vi "Set PublicEvents.vi"(8 "error in (no error)":errorcluster, 10 "Public Events":T1, 11 "DbgTimers in":refnum<class "DbgTimers.lvclass">) -> (0 "error out":errorcluster, 3 "DbgTimers out":refnum<class "DbgTimers.lvclass">)   [LabVIEW 2017, in "DbgTimers.lvclass"]
doc: "Developed by Kevin Thompson\nkevin@thompsonengineering.net\n\nCopyright 2018-2020\nThompson Engineering, LLC"
uses:
  DbgTimers.lvclass
  DataTypes/Public Events--cluster.ctl
  Ichor_Common/DataTypes/TD Async CmdMsg EventData--cluster.ctl
  DbgTimers.lvclass/DbgTimers.ctl
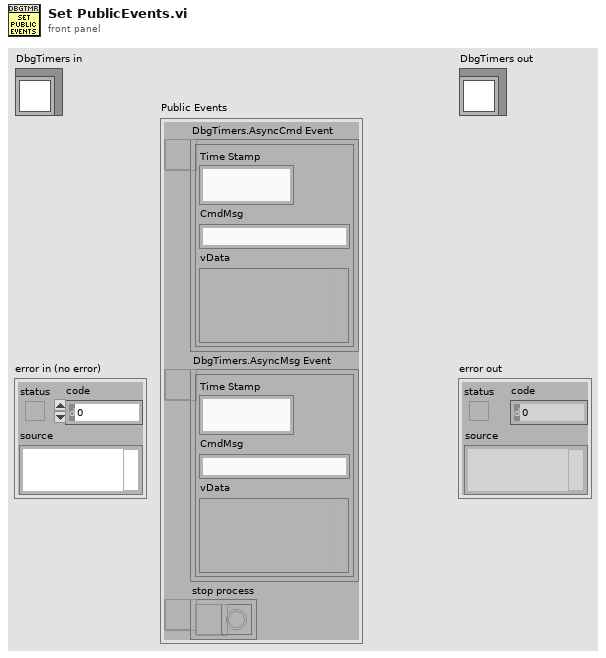
[diagram p1: front panel]
types:
  T1 = typedef "DbgTimers.lvclass/Public Events--cluster.ctl" = cluster{"DbgTimers.AsyncCmd Event":refnum<user-event>, "DbgTimers.AsyncMsg Event":refnum<user-event>, "stop process":refnum<user-event>}
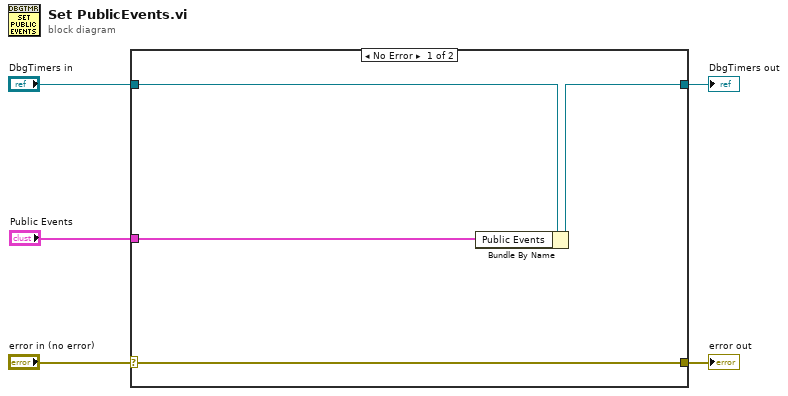
[diagram p0: block diagram]
diagram:
  n1 = case shown="No Error" "error in (no error)" {
    selector: "error in (no error)" -> [w9 w10]
    tunnel: [w9 w10] -> w4
    tunnel: [w7 w11] -> w2
    tunnel: "DbgTimers in" -> [w8 w11]
    tunnel: "Public Events" -> [w6 _]
    frame No Error {
      n2 = Bundle By Name(cluster=w8, "Public Events"=w6) -> (w7:refnum<class "DbgTimers.lvclass">)
    }
    frame Error {
    }
  }
  "error out" <- w4
  "DbgTimers out" <- w2
